vi "TestStand, NumericLimitTest, Set Limits.vi"(8 "error in":errorcluster, 10 "CDT_type":T1={"Measurement Name"="Signal_1", "Result"=3.0, "Low Limit"=-100.0, "High Limit"=100.0, "Units"="nA", "Comp"="GELE", "DataFmt"="%.3f", "LimitFmt"="%.3f"} {"Result" format="%.3g"; "High Limit" format="%.3g"; "Low Limit" format="%.3g"}, 11 "Sequence Context":refnum<k7>) -> (0 "error out":errorcluster, 3 "Sequence Context dup":refnum<k7>)   [LabVIEW 2010]
doc: "Sets TestStand Multiple Numeric Test properties for the following:\n\nRunState.Step.\nRunState.Step.Limits.High\nRunState.Step.Limits.Low\nRunState.Step.Result.Units\nRunState.Step.Result.Comp"
uses:
  TestStand_Result Control.ctl
  <vilib>/addons/TestStand/_TSUtility.llb/TestStand - Get Property Value (Object).vi
  <vilib>/addons/TestStand/_TSUtility.llb/TestStand - Set Property Value (String).vi
  <vilib>/addons/TestStand/_TSUtility.llb/TestStand - Set Property Value (Number).vi
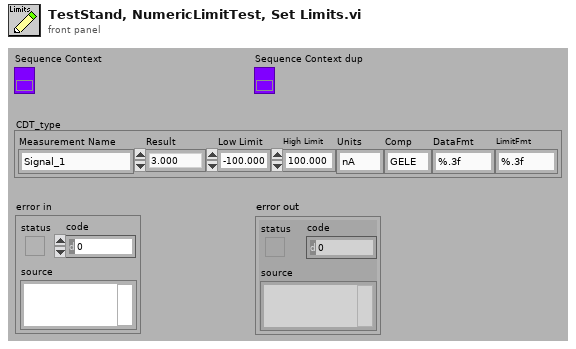
[diagram p1: front panel]
types:
  T1 = typedef "TestStand_Result Control.ctl" = cluster{"Measurement Name":string, "Result":dbl, "Low Limit":dbl, "High Limit":dbl, "Units":string, "Comp":string, "DataFmt":string, "LimitFmt":string}
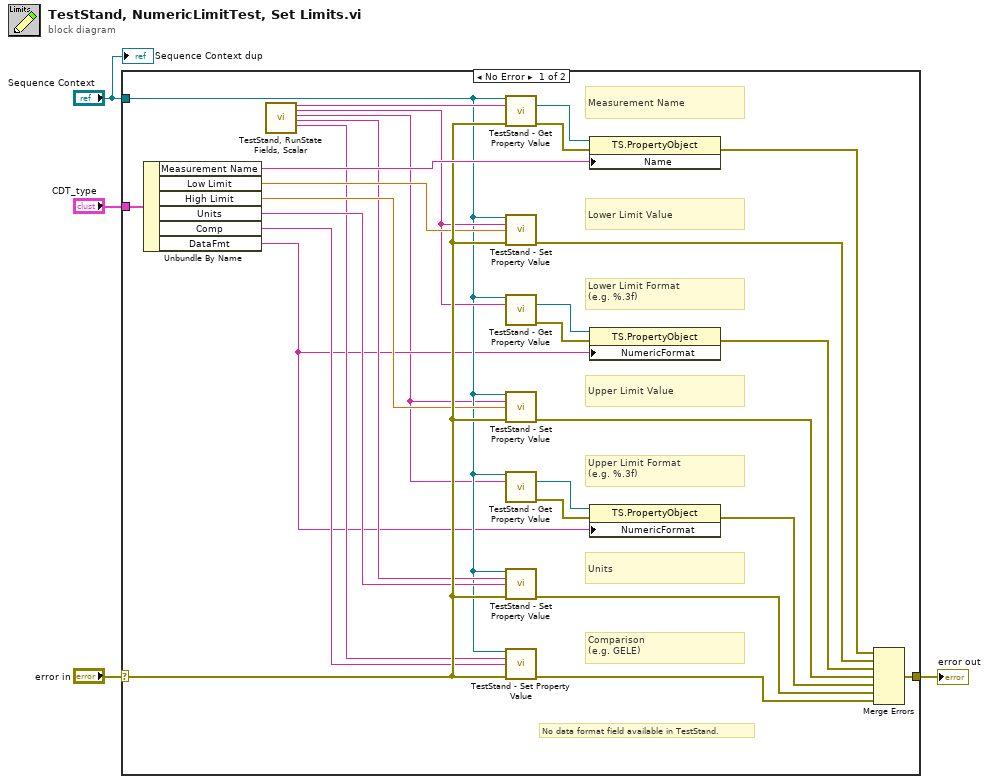
[diagram p0: block diagram]
diagram:
  n1 = case shown="No Error" "error in" {
    selector: "error in" -> [w25 w33]
    tunnel: [w27 w33] -> w4
    tunnel: "Sequence Context" -> [w11 _]
    tunnel: "CDT_type" -> [w26 _]
    frame No Error {
      # "No data format field available in TestStand."
      # "Comparison\n(e.g. GELE)"
      # "Units"
      # "Upper Limit Format\n(e.g. %.3f)"
      # "Upper Limit Value"
      # "Lower Limit Format\n(e.g. %.3f)"
      # "Lower Limit Value"
      # "Measurement Name"
      n2 = Unbundle By Name(w26) -> ("Measurement Name"=w32:string, "Low Limit"=w24:dbl, "High Limit"=w23:dbl, "Units"=w22:string, "Comp"=w21:string, "DataFmt"=w10:string)
      n3 = call "TestStand, RunState Fields, Scalar.vi"() -> ("Measurement Name"=w20:string, "Low Limit"=w15:string, "High Limit"=w9:string, "Units"=w19:string, "Comp"=w18:string)  [unwired: 15 in]
      n4 = call-poly <vilib>:"TestStand - Get Property Value.vi"("Sequence Context In"=w11, "Lookup String"=w20, "error in (no error)"=w25) -> ("Value"=w8:refnum<k7>, "error out"=w7:errorcluster)  [unwired: 10 in, 1 out]
      n5 = call-poly <vilib>:"TestStand - Set Property Value.vi"("Sequence Context In"=w11, "Lookup String"=w15, "New Value"=w24, "error in (no error)"=w25) -> ("error out"=w31:errorcluster)  [unwired: 10 in, 1 out]
      n6 = call-poly <vilib>:"TestStand - Get Property Value.vi"("Sequence Context In"=w11, "Lookup String"=w15) -> ("Value"=w17:refnum<k7>, "error out"=w16:errorcluster)  [unwired: 11 in, 1 out]
      n7 = call-poly <vilib>:"TestStand - Set Property Value.vi"("Sequence Context In"=w11, "Lookup String"=w9, "New Value"=w23, "error in (no error)"=w25) -> ("error out"=w28:errorcluster)  [unwired: 10 in, 1 out]
      n8 = call-poly <vilib>:"TestStand - Get Property Value.vi"("Sequence Context In"=w11, "Lookup String"=w9) -> ("Value"=w6:refnum<k7>, "error out"=w13:errorcluster)  [unwired: 11 in, 1 out]
      n9 = call-poly <vilib>:"TestStand - Set Property Value.vi"("Sequence Context In"=w11, "Lookup String"=w19, "New Value"=w22, "error in (no error)"=w25) -> ("error out"=w29:errorcluster)  [unwired: 10 in, 1 out]
      n10 = call-poly <vilib>:"TestStand - Set Property Value.vi"("Sequence Context In"=w11, "Lookup String"=w18, "New Value"=w21, "error in (no error)"=w25) -> ("error out"=w30:errorcluster)  [unwired: 10 in, 1 out]
      n11 = property class="TS.PropertyObject"(reference=w8, error in=w7, "Name"=w32) -> (error out=w5:errorcluster)  [unwired: 1 out]
      n12 = property class="TS.PropertyObject"(reference=w17, error in=w16, "NumericFormat"=w10) -> (error out=w14:errorcluster)  [unwired: 1 out]
      n13 = property class="TS.PropertyObject"(reference=w6, error in=w13, "NumericFormat"=w10) -> (error out=w12:errorcluster)  [unwired: 1 out]
      n14 = Merge Errors(w5, w31, w14, w28, w12, w29, w30) -> (w27:errorcluster)
    }
    frame Error {
    }
  }
  "error out" <- w4
  "Sequence Context dup" <- "Sequence Context"
